vi "test.vi"() -> ()   [LabVIEW 2015]
panel:
  out "subarray 2":dbl[](array[numeric])
  out "subarray":dbl[](array[numeric])
  out "XY Graph":cluster{dbl[], dbl[]}(graph)
  out "standard output 4":string
  out "standard error 4":string
  out "concatenated string 2":string
  out "standard output 5":string
  out "standard error 5":string
  out "concatenated string 3":string
  out "concatenated string 7":string
  out "standard output 7":string
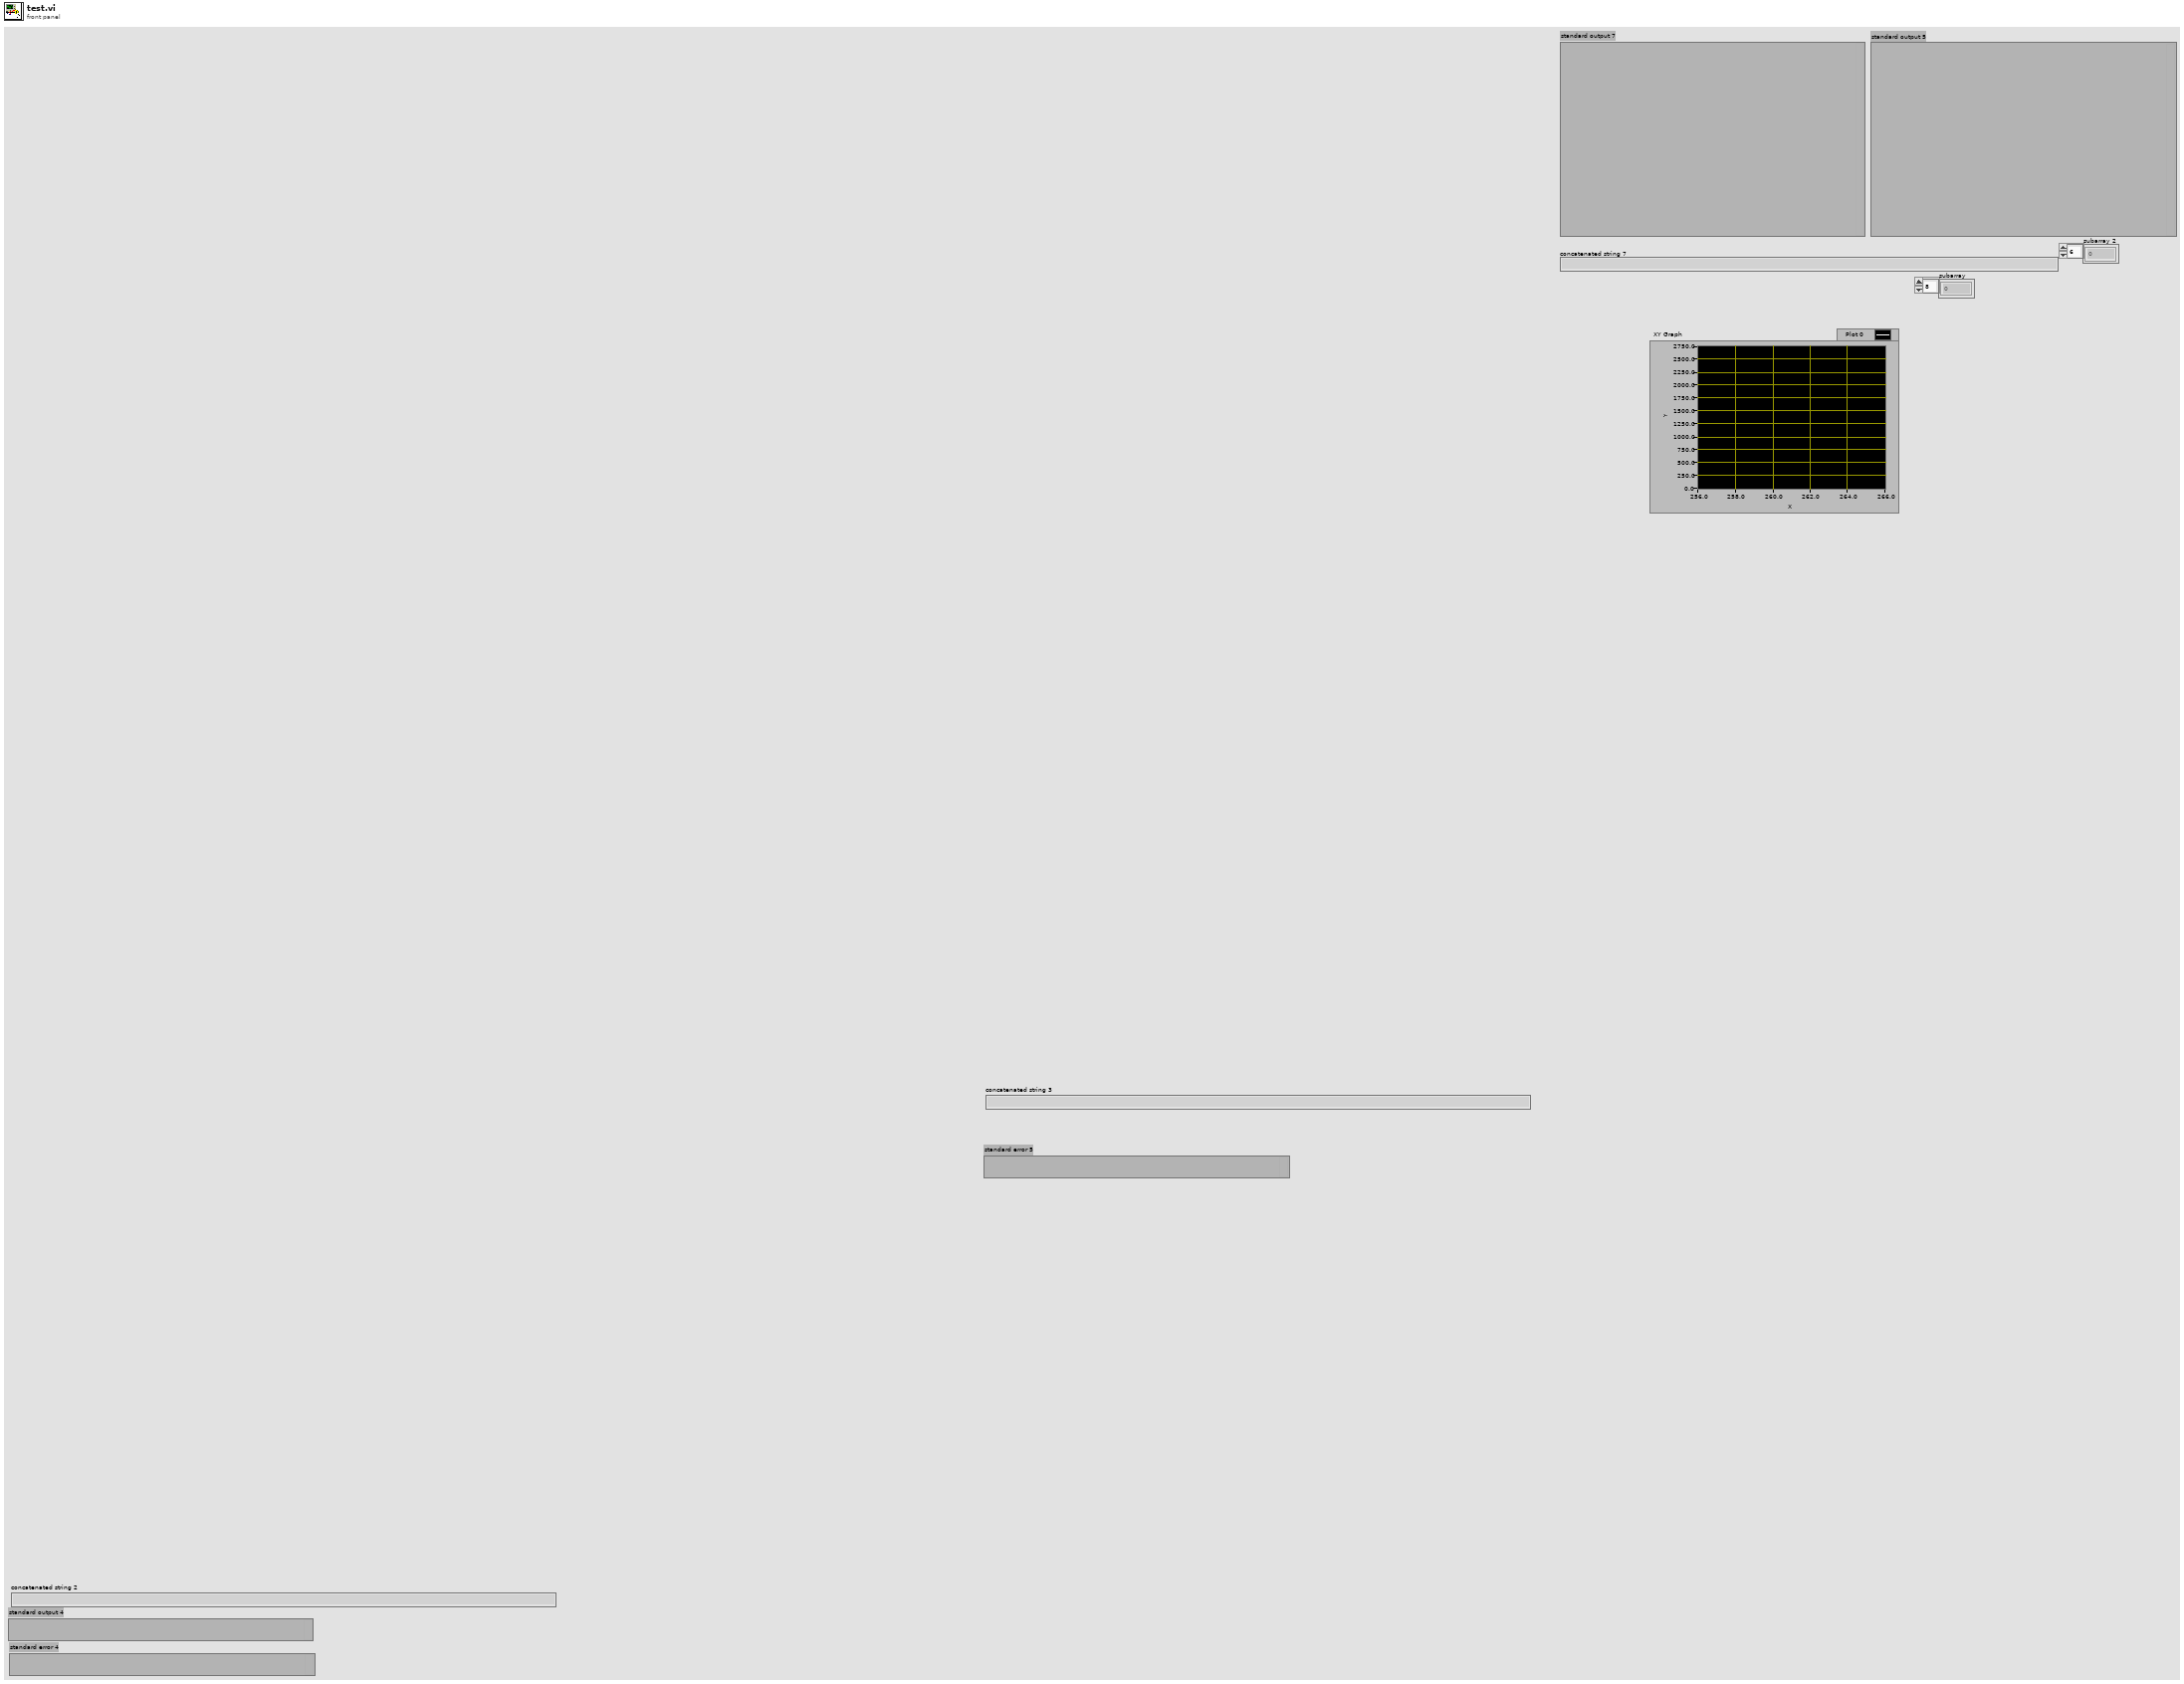
[diagram p1: front panel]
types:
  T1 = typedef "imagedata.ctl" = cluster{"image type":i32, "image depth":i32, "image":u8[], "mask":u8[], "colors":u32[], "Rectangle":cluster{"left":i16, "top":i16, "right":i16, "bottom":i16}}
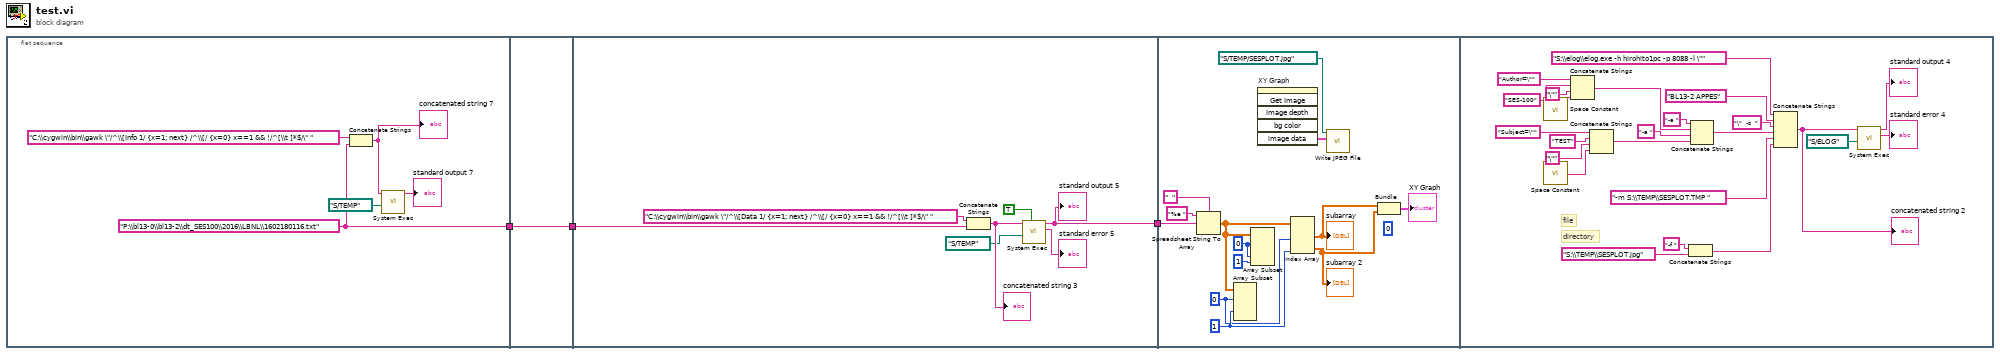
[diagram p0: block diagram]
diagram:
  n1 = flat-sequence {
    tunnel: [w5] -> w3
    tunnel: w3 -> [w9]
    tunnel: [w9] -> w2
    tunnel: w2 -> [w12]
    tunnel: [w10] -> w1
    tunnel: w1 -> [w28]
    frame #0 {
      w5 = "P:\\bl13-0\\bl13-2\\dt_SES100\\2016\\LBNL\\1602180116.txt" ("string")
      n2 = Concatenate Strings("C:\\cygwin\\bin\\gawk \"/^\\[Info 1/ {x=1; next} /^\\[/ {x=0} x==1 && !/^[\\t ]*$/\" " ("command line"), w5) -> (w6:string)
      "concatenated string 7" <- w6
      n3 = call <vilib>:"System Exec.vi"("working directory"=path "S:/TEMP", "command line"=w6) -> ("standard output"=→"standard output 7":string)  [unwired: 6 in, 3 out]
    }
    frame #1 {
    }
    frame #2 {
      n4 = Concatenate Strings("C:\\cygwin\\bin\\gawk \"/^\\[Data 1/ {x=1; next} /^\\[/ {x=0} x==1 && !/^[\\t ]*$/\" " ("command line"), w12) -> (w16:string)
      "concatenated string 3" <- w16
      n5 = call <vilib>:"System Exec.vi"("wait until completion? (T)"=TRUE, "working directory"=path "S:/TEMP", "command line"=w16) -> ("standard error"=→"standard error 5":string, "standard output"=w10:string)  [unwired: 5 in, 2 out]
      "standard output 5" <- w10
    }
    frame #3 {
      (unwired) 0 ("index")
      w23 = 1 ("index")
      w22 = 0 ("index")
      w26 = 0 ("index")
      n6 = Spreadsheet String To Array(delimiter (Tab)="  " ("format string"), format string="%e ", spreadsheet string=w28) -> (array=w24:dbl[][])  [unwired: 1 in]
      n7 = Array Subset(array=w24, index (row)=w22, index (col)=w23) -> ()  [unwired: 2 in, 1 out]
      n8 = Array Subset(array=w24, index (row)=w26, index (col)=w26, length (col)=1 ("index")) -> ()  [unwired: 1 in, 1 out]
      n9 = invoke on="XY Graph" class="XYGraph (strict)" method="Get Image"() -> ("image data"=w18:T1)  [unwired: 6 in, 5 out]
      n10 = Index Array(array=w24, index (col) #1=w22, index (col) #2=w23) -> (element #1=w21:dbl[], element #2=w20:dbl[])  [unwired: 2 in]
      "subarray" <- w21
      "subarray 2" <- w20
      n11 = call <vilib>:"Write JPEG File.vi"("image data"=w18, "path to JPEG file"=path "S:/TEMP/SESPLOT.jpg" ("file path (use dialog)")) -> ()  [unwired: 8 in, 2 out]
      n12 = Bundle(w21, w20) -> (→"XY Graph":cluster{dbl[], dbl[]})  [unwired: 1 in]
    }
    frame #4 {
      # "file"
      # "directory"
      n13 = call <vilib>:"Space Constant.vi"() -> ("String"=w39:string)
      n14 = call <vilib>:"Space Constant.vi"() -> ("String"=w40:string)
      n15 = Concatenate Strings("Author=\"" ("string"), "SES-100", "\"" ("string"), w39) -> (w37:string)
      n16 = Concatenate Strings("Subject=\"" ("string"), "TEST" ("string"), "\"" ("string"), w40) -> (w35:string)
      n17 = Concatenate Strings("-f " ("string"), "S:\\TEMP\\SESPLOT.jpg" ("string")) -> (w32:string)
      n18 = Concatenate Strings("-a ", w37, "-a " ("string"), w35) -> (w36:string)
      n19 = Concatenate Strings("S:\\elog\\elog.exe -h hirohito1pc -p 8088 -l \"" ("command line"), "BL13-2 APPES", "\"  -s  " ("command line"), w36, "-m S:\\TEMP\\SESPLOT.TMP " ("string"), w32) -> (w48:string)
      "concatenated string 2" <- w48
      n20 = call <vilib>:"System Exec.vi"("working directory"=path "S:/ELOG", "command line"=w48) -> ("standard error"=→"standard error 4":string, "standard output"=→"standard output 4":string)  [unwired: 6 in, 2 out]
    }
  }
